vi "CmdShell.vi"(9 "Command Line                     Standard Input":string[][](array[string])=[["cmd", "attrib -r *.dat \n"], ["cmd", "attrib -r *.cfg \n"]], 11 "working directory":path=path "c:/emcore/programs/data") -> (0 "Error":errorcluster[](array[cluster]), 1 "Return Code":i32[](array[numeric]), 2 "Standard Error":string[](array[string]), 3 "Standard Output":string[](array[string]), 4 "All OK":bool)   [LabVIEW 2011]
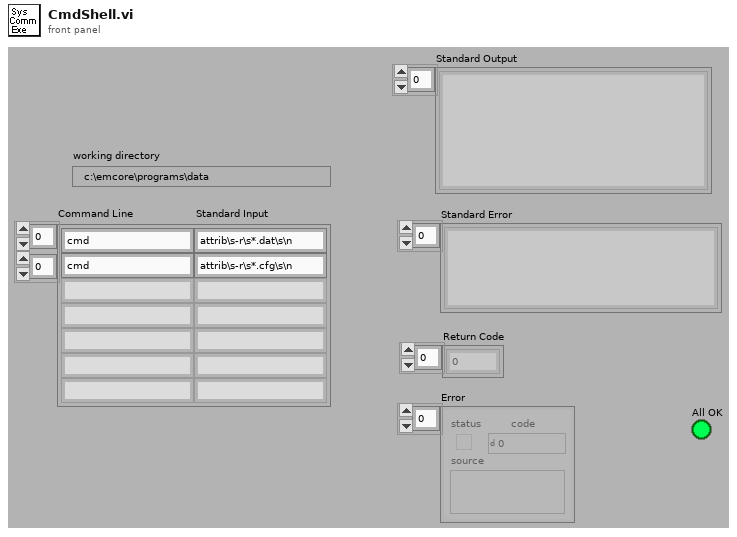
[diagram p1: front panel]
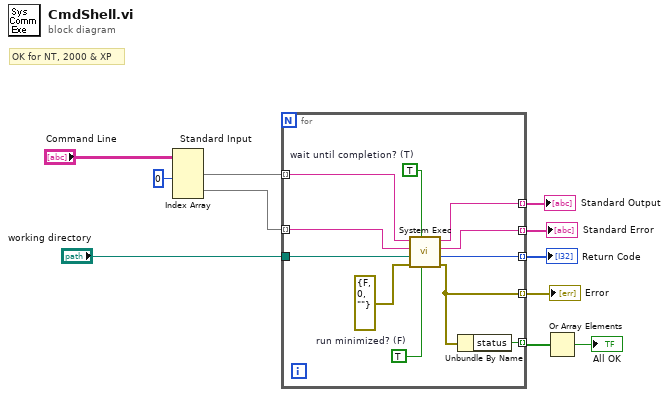
[diagram p0: block diagram]
diagram:
  # "OK for NT, 2000 & XP"
  n1 = Index Array(array="Command Line                     Standard Input", index (col) #1=0 ("Disabled Index (col)")) -> (element #1=w4:string[], element #2=w1:string[])  [unwired: 3 in]
  n2 = for {
    tunnel: w1 -> [w22] mode=indexing
    tunnel: w4 -> [w20] mode=indexing
    tunnel: "working directory" -> [w17]
    tunnel: [w16] -> w9 mode=indexing
    tunnel: [w12] -> w10 mode=indexing
    tunnel: [w15] -> w11 mode=indexing
    tunnel: [w14] -> w7 mode=indexing
    tunnel: [w13] -> w3 mode=indexing
    w19 = TRUE  # run minimized? (F)
    w21 = TRUE  # wait until completion? (T)
    n3 = call <vilib>:"System Exec.vi"("run minimized? (F)"=w19, "wait until completion? (T)"=w21, "error in (no error)"=errorcluster {"status"=FALSE, "code"=0, "source"=""}, "working directory"=w17, "standard input"=w22, "command line"=w20) -> ("error out"=w14:errorcluster, "return code"=w16:i32, "standard error"=w12:string, "standard output"=w15:string)  [unwired: 2 in]
    n4 = Unbundle By Name(w14) -> ("status"=w13:bool)
  }
  "Standard Output" <- w11
  "Standard Error" <- w10
  "Return Code" <- w9
  "Error" <- w7
  n5 = Or Array Elements(Boolean array=w3) -> (logical OR=→"All OK":bool)
